vi "EXPRES Receive Message.vi"(8 "error in (no error)":errorcluster, 11 "TCP Network Connection in":refnum<k5>) -> (0 "error out":errorcluster, 1 "JSON string":string, 2 "method":string, 3 "connection ID out":refnum<k5>)   [LabVIEW 2016]
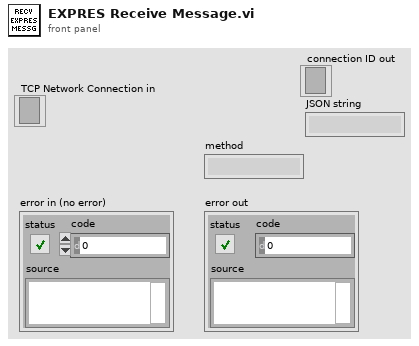
[diagram p1: front panel]
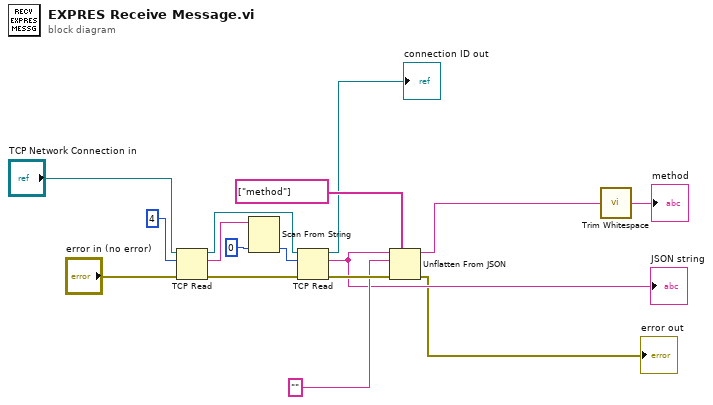
[diagram p0: block diagram]
diagram:
  n1 = TCP Read(connection ID="TCP Network Connection in", bytes to read=4, error in (no error)="error in (no error)") -> (connection ID out=w10:refnum<k5>, data out=w7:string, error out=w9:errorcluster)  [unwired: 2 in]
  n2 = Scan From String(input string=w7, default 1=0) -> (output 1=w11:i32)  [unwired: 3 in, 3 out]
  n3 = TCP Read(connection ID=w10, bytes to read=w11, error in (no error)=w9) -> (connection ID out=→"connection ID out":refnum<k5>, data out=w2:string, error out=w14:errorcluster)  [unwired: 2 in]
  "JSON string" <- w2
  n4 = Unflatten From JSON(path=string[] ["method"], JSON string=w2, type and defaults="", error in (no error)=w14) -> (value=w15:string, error out=→"error out":errorcluster)  [unwired: 3 in]
  n5 = call <vilib>:"Trim Whitespace.vi"("string"=w15) -> ("trimmed string"=→"method":string)  [unwired: 1 in]
